vi "PMBus Hard Init.vi"(6 "OwnAddr":u8, 7 "ClockSpeed":u32, 9 "PMBusIndex":i32, 10 "DevIndex":i32, 11 "DevType":i32) -> (3 "function return":i32)   [LabVIEW 2010, in "ControlPMBus.lvlib"]
doc: "int WINAPI PMBus_HardInit(int DevType,int DevIndex,int PMBusIndex,unsigned int ClockSpeed, unsigned char OwnAddr);"
uses:
  ControlPMBus.lvlib
  ControlPMBus/Ginkgo_Driver.dll
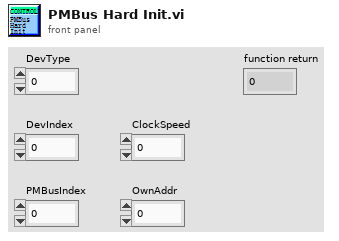
[diagram p1: front panel]
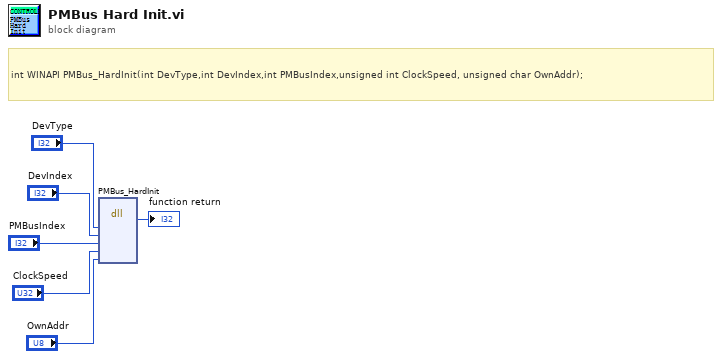
[diagram p0: block diagram]
diagram:
  # "int WINAPI PMBus_HardInit(int DevType,int DevIndex,int PMBusIndex,unsigned int ClockSpeed, unsigned char OwnAddr);"
  n1 = dll-call lib="E:/Project/vt_ginkgo/truck/Ginkgo Driver/vs2010/Ginkgo_USB-I2C&SPI&CAN_API_v2.0.3.3/lib/labview_32bit/ControlPMBus/Ginkgo_Driver.*" fn="PMBus_HardInit"("DevType"="DevType", "DevIndex"="DevIndex", "PMBusIndex"="PMBusIndex", "ClockSpeed"="ClockSpeed", "OwnAddr"="OwnAddr") -> (→"function return":i32)  [unwired: 8 in, 2 out]
